vi "Destroy.vi"(8 "error in (no error)":errorcluster, 11 "Plugin Manager in":refnum<class "CIFPluginLoader.lvclass">) -> (0 "error out":errorcluster, 3 "Plugin Manager out":refnum<class "CIFPluginLoader.lvclass">)   [LabVIEW 2021, in "CIFPluginLoader.lvclass"]
uses:
  CIFPluginLoader.lvclass
  CIFPluginLoader.lvclass/CIFPluginLoader.ctl
  CIFUtilities/CIFLogs/Typedef/Message Type.ctl
  typedef/Loaded Plugin Map.ctl
  <vilib>/gRPC/LabVIEW gRPC Servicer/ServiceBase/ServiceBase.lvclass
  CIFUtilities/CIFLogs/CIFLogs.lvlib
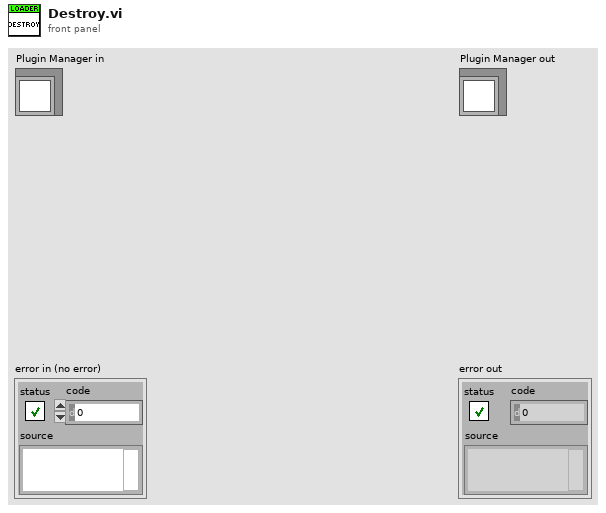
[diagram p1: front panel]
types:
  T1 = typedef "CIFLogs.lvlib/Message Type.ctl" = enum16{"Error", "Information", "Print Terminal", "Configuration"}
  T2 = typedef "CIFPluginLoader.lvclass/Loaded Plugin Map.ctl" = map{string, refnum<vi>}
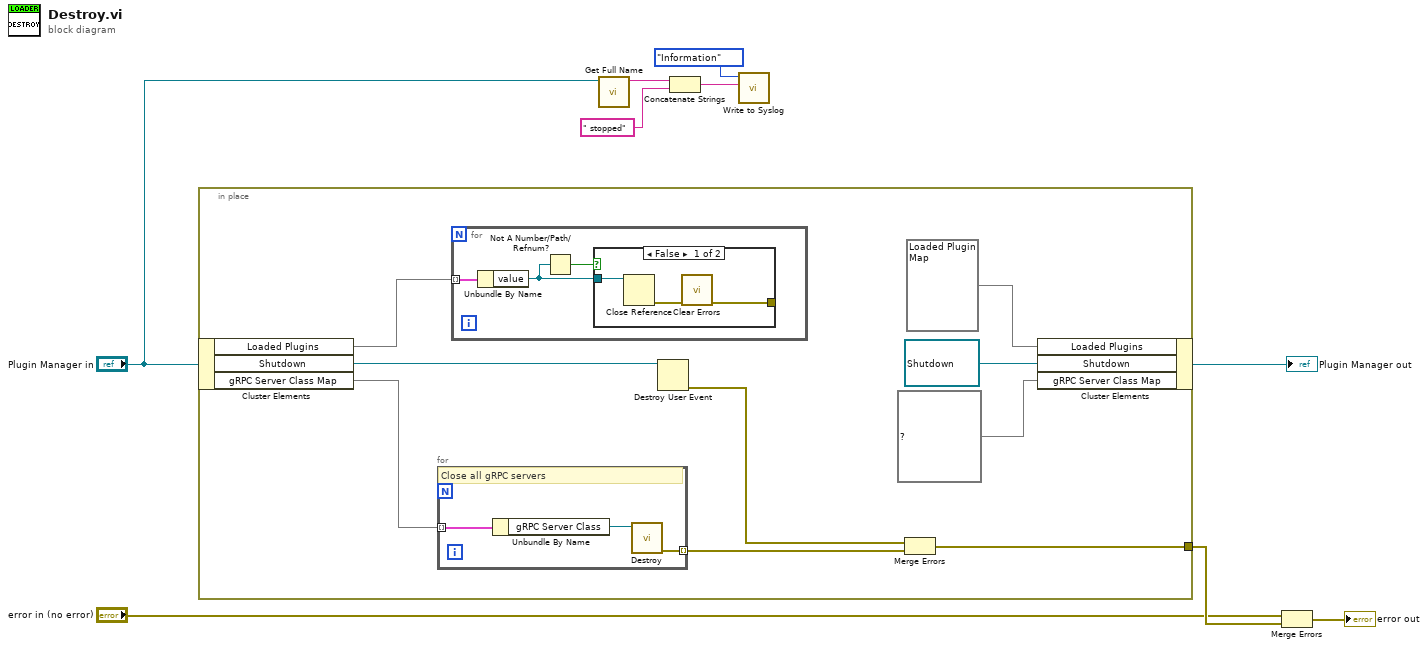
[diagram p0: block diagram]
diagram:
  n1 = in-place {
    in-place-border: [w15] -> w8
    n2 = in-place-cluster #1("Plugin Manager in") -> ("Loaded Plugins"=w11:T2, "Shutdown"=w14:refnum<user-event>, "gRPC Server Class Map"=w18:map{string, refnum<class "ServiceBase.lvclass">})
    n3 = for {
      tunnel: w18 -> [w27] mode=indexing
      tunnel: [w25] -> w16 mode=indexing
      # "Close all gRPC servers"
      n4 = Unbundle By Name(w27) -> ("gRPC Server Class"=w26:refnum<class "ServiceBase.lvclass">)
      n5 = call-dynamic "Destroy.vi"("SignalGeneratorService in"=w26) -> ("error out"=w25:errorcluster)  [unwired: 9 in, 1 out]
    }
    n6 = for {
      tunnel: w11 -> [w20] mode=indexing
      n7 = Unbundle By Name(w20) -> ("value"=w19:refnum<vi>)
      n8 = Not A Number/Path/Refnum?(number/path/refnum=w19) -> (NaN/Path/Refnum?=w21:bool)
      n9 = case shown="False" w21 {
        tunnel: w19 -> [w24 _]
        tunnel: [w22 _] -> _
        frame False {
          n10 = Close Reference(reference=w24) -> (error out=w23:errorcluster)  [unwired: 1 in]
          n11 = call <vilib>:"Clear Errors.vi"("error in (no error)"=w23) -> ("error out"=w22:errorcluster)  [unwired: 5 in, 1 out]
        }
        frame True {
        }
      }
    }
    n12 = Destroy User Event(user event=w14) -> (error out=w13:errorcluster)  [unwired: 1 in]
    n13 = Merge Errors(w13, w16) -> (w15:errorcluster)
    n14 = in-place-cluster #1("Loaded Plugins"=T2 {}, "Shutdown"=refnum<user-event> refnum ("Parallel Events.Shutdown"), "gRPC Server Class Map"=map{string, refnum<class "ServiceBase.lvclass">} {}) -> (→"Plugin Manager out":refnum<class "CIFPluginLoader.lvclass">)
  }
  n15 = call "Get Full Name.vi"("CIFPluginLoader in"="Plugin Manager in") -> ("Full Name"=w2:string)  [unwired: 10 in]
  n16 = Concatenate Strings(w2, " stopped" ("message")) -> (w3:string)
  n17 = call "Write to Syslog.vi"("message"=w3, "CIF Message Type"=Message_Type."Information") -> ()  [unwired: 9 in, 1 out]
  n18 = Merge Errors("error in (no error)", w8) -> (→"error out":errorcluster)
